vi "Log in dialog.vi"(0 "Enable":bool=TRUE, 5 "error in (no error)":errorcluster) -> (16 "Password":string, 17 "ID":string, 18 "OK":bool, 19 "error out":errorcluster)   [LabVIEW 2017]
doc: "Displays a standard dialog box that prompts users to enter information, such as a user name and password.\n--------------------\n\nThis Express VI is configured as follows:\n\nMessage to Display to the User:\nThe inputs are: \nText Entry Box: ID\nText Entry Box: Password"
panel:
  in  "Password":string
  in  "ID":string
  out "String":string
  in  "Cancel":bool
  in  "OK2":bool
  in  "OK1":bool
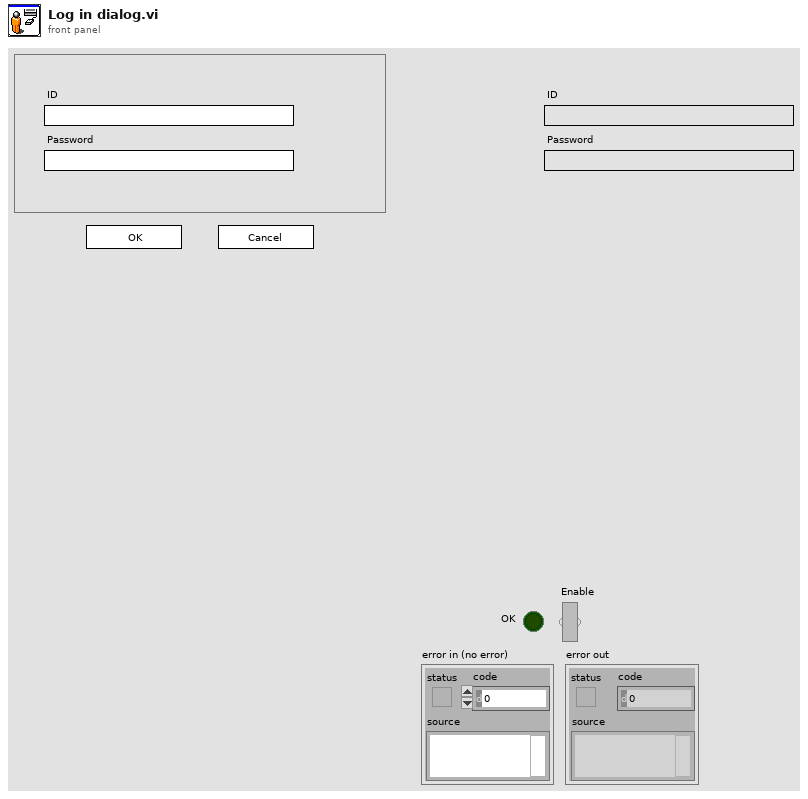
[diagram p1: front panel]
types:
  T1 = cluster{"Input Name":string, "Input Data Type":i32}[]
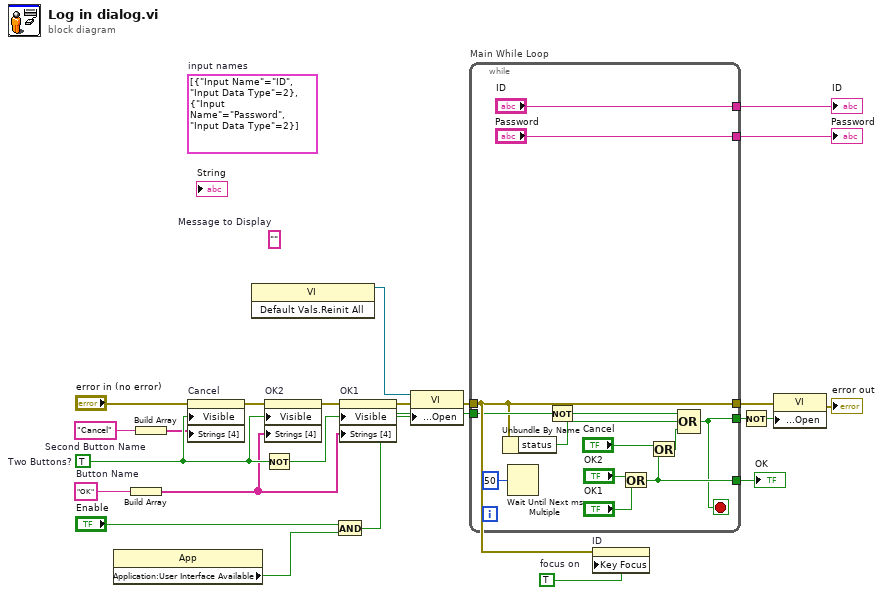
[diagram p0: block diagram]
diagram:
  w3 = TRUE  # focus on
  (unwired) T1 [{"Input Name"="ID", "Input Data Type"=2}, {"Input Name"="Password", "Input Data Type"=2}]  # input names
  w15 = "Cancel"  # Second Button Name
  w13 = "OK"  # Button Name
  (unwired) ""  # Message to Display
  w23 = TRUE  # Two Buttons?
  n1 = property class="App"() -> ("Application:User Interface Available"=w5:bool)  [unwired: 2 in, 2 out]
  n2 = Build Array(w13) -> (w14:string[])
  n3 = Build Array(w15) -> (w16:string[])
  n4 = property on="Cancel" class="Bool"(error in="error in (no error)", "Visible"=w23, "Strings [4]"=w16) -> (error out=w20:errorcluster)  [unwired: 1 in, 1 out]
  n5 = invoke class="VI" method="Default Vals.Reinit All"() -> (reference out=w4:refnum<vi>)  [unwired: 3 in, 2 out]
  n6 = Not(x=w23) -> (.not. x?=w21:bool)
  n7 = property on="OK2" class="Bool"(error in=w20, "Visible"=w23, "Strings [4]"=w14) -> (error out=w19:errorcluster)  [unwired: 1 in, 1 out]
  n8 = And(x="Enable", y=w5) -> (x .and. y?=w6:bool)
  n9 = property on="OK1" class="Bool"(error in=w19, "Visible"=w21, "Strings [4]"=w14) -> (error out=w12:errorcluster)  [unwired: 1 in, 1 out]
  n10 = property class="VI"(reference=w4, error in=w12, "Front Panel Window:Open"=w6) -> (error out=w11:errorcluster)  [unwired: 1 out]
  n11 = while "Main While Loop" {
    tunnel: [w33] -> w22
    tunnel: w6 -> [w31]
    tunnel: [w29] -> w17
    tunnel: w11 -> [w28]
    tunnel: [w28] -> w9
    tunnel: ["ID"] -> w2
    tunnel: ["Password"] -> w1
    stop <- w29 stop-if-true
    n12 = Unbundle By Name(w28) -> ("status"=w26:bool)
    n13 = Wait Until Next ms Multiple(millisecond multiple=u32 50) -> ()  [unwired: 1 out]
    n14 = Not(x=w31) -> (.not. x?=w30:bool)
    n15 = Or(x="OK2", y="OK1") -> (x .or. y?=w33:bool)
    n16 = Or(x="Cancel", y=w33) -> (x .or. y?=w27:bool)
    n17 = Compound Arithmetic op=OR(w30, w26, w27) -> (w29:bool)
  }
  "OK" <- w22
  "ID" <- w2
  "Password" <- w1
  n18 = property on="ID" class="Str"(error in=w11, "Key Focus"=w3) -> ()  [unwired: 1 in, 2 out]
  n19 = Not(x=w17) -> (.not. x?=w18:bool)
  n20 = property class="VI"(error in=w9, "Front Panel Window:Open"=w18) -> (error out=→"error out":errorcluster)  [unwired: 1 in, 1 out]
